vi "Transfer Image Pixel Data To Host x8.vi"(0 "image pixel data":u8[](array[numeric]), 1 "reset":bool, 2 "image pixel data dma fifo x8":refnum<k21>, 9 "input valid":bool) -> (4 "overflow":bool, 14 "ready for input":bool)   [LabVIEW 2020, in "GettingStarted_Common_148X_FPGA.lvlib"]
uses:
  GettingStarted_Common_148X_FPGA.lvlib
  <vilib>/rvi/DataTransferAndStorage/Container/Common/niFpgaContainerExecOnDevCompGetState.vi
  <vilib>/rvi/Emulation/niFpgaSctlEmulationGetInTimedLoop.vi
  <vilib>/rvi/errors/niFpgaSetErrorForExecOnDevCompSimple.vi
  <vilib>/rvi/eio/common/nirviEmuReportErrorAndStop.vi
  <vilib>/rvi/interface/RandomDataEmulation/nirviRandomDataAcquireLock.vi
  <vilib>/rvi/interface/RandomDataEmulation/nirviRandomDataQueueStore.vi
  <vilib>/rvi/interface/RandomDataEmulation/nirviRandomDataReleaseLock.vi
  <vilib>/rvi/interface/RandomDataEmulation/nirviFPGAContextMergeError.vi
  <vilib>/rvi/interface/RandomDataEmulation/nirviRandomDataCheckExitLoopConditions.vi
  <vilib>/express/rvi/timingcommon/nirviCommon.vi
  <vilib>/rvi/interface/RandomDataEmulation/niFpgaRandomDataHandleErrors.vi
  <vilib>/rvi/DataTransferAndStorage/Container/XNode/niFpgaContainer.xnode
  <vilib>/rvi/FIFO/Fifo_Resource/niFpgaFifoEmulationRefInMultiElement.vi
  <instrlib>/_niInstr/Basic Elements/v1/FPGA/niInstr Basic Elements v1 FPGA.lvlib
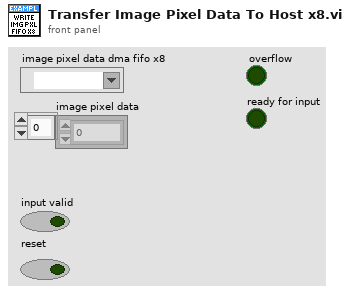
[diagram p1: front panel]
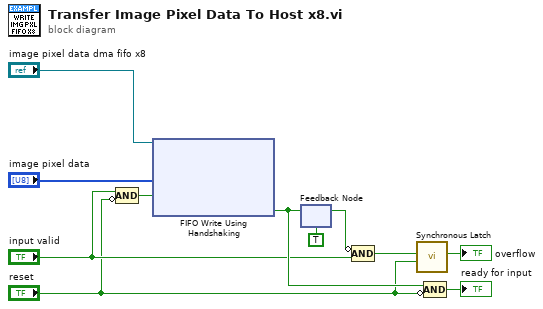
[diagram p0: block diagram]
diagram:
  n1 = Compound Arithmetic op=AND("input valid", invert "reset") -> (w1:bool)
  n2 = xnode ("FIFO Write Using Handshaking")("Element"="image pixel data", "Input Valid"=w1, "FIFO In"="image pixel data dma fifo x8") -> ("Ready for Input"=w6:bool)  [unwired: 1 out]
  n3 = feedback #1(TRUE ("Ready for Input")) -> (w8:bool)
  n4 = feedback-in #1(w6) -> ()
  n5 = Compound Arithmetic op=AND(invert w8, "input valid") -> (w11:bool)
  n6 = call <instrlib>:"Synchronous Latch.vi"("clear"="reset", "set"=w11) -> ("out"=→"overflow":bool)  [unwired: 9 in]
  n7 = Compound Arithmetic op=AND(w6, invert "reset") -> (→"ready for input":bool)
